vi "IviTriggerToProperty.vi"(8 "error in (no error)":errorcluster, 11 "IVI_Class.lvclass":refnum<class "IVI_Class.lvclass">) -> (0 "error out":errorcluster, 3 "IVI_Class.lvclass":refnum<class "IVI_Class.lvclass">)   [LabVIEW 2018, in "ScopePlugins.lvlib" / "IVI_Class.lvclass"]
doc: "Reads IVI Scope Acquisition properties and writes them into the Scope class Acquisition Properties"
uses:
  IVI_Class.lvclass
  C:/Users/ico/Documents/Projects/NistPluggableModules/Scope/ScopePlugins/ScopePluginBaseClass/ScopePluginsBase.lvclass
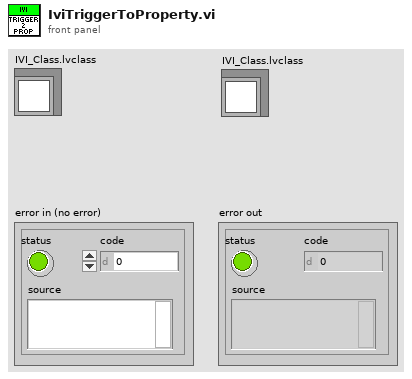
[diagram p1: front panel]
types:
  T1 = typedef "ScopePlugins.lvlib/ScopePluginsBase.lvclass/TriggerSettings.ctl" = cluster{"Common Trigger Settings":cluster{"Trigger Delay":dbl, "Reference Position":dbl, "Trigger Modifier":i32, "Auto Triggered":bool}, "Specific Trigger Settings":cluster{"Source":string, "Holdoff":dbl, "Level":dbl, "Trigger Slope":enum16{"Negative", "Positive"}, "Type":enum16{"Immediate", "Edge", "Digitial", "Window", "Hysteresis", "Width", "Runt", "Glitch", "TV", "AC Line"}, "Window Mode":i32, "Low Level":dbl, "High Level":dbl, "Coupling":u16, "Hysteresis":dbl}}
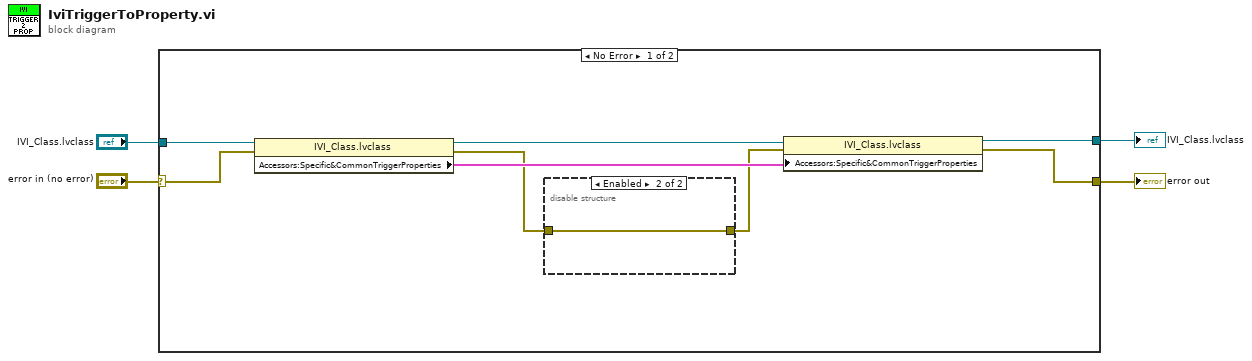
[diagram p0: block diagram]
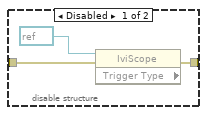
[diagram p2: hidden frame]
diagram:
  n1 = case shown="No Error" "error in (no error)" {
    selector: "error in (no error)" -> [w10 w17]
    tunnel: "IVI_Class.lvclass" -> [w12 w18]
    tunnel: [w11 w18] -> w3
    tunnel: [w9 w17] -> w1
    frame No Error {
      n2 = property class="IVI_Class.lvclass"(reference=w12, error in=w10) -> (reference out=w7:refnum<class "IVI_Class.lvclass">, error out=w6:errorcluster, "Accessors:Specific&CommonTriggerProperties"=w8:T1)
      n3 = disable-structure shown="Enabled" {
        disable-tunnel: [w15 w16] -> w5
        disable-tunnel: w6 -> [w13 w16]
        frame Disabled {
          n4 = property class="IviScope" props=["Trigger Type"](reference=refnum<k15> refnum ("reference out"), error in=w13) -> (error out=w15:errorcluster)  [unwired: 2 out]
        }
        frame Enabled {
        }
      }
      n5 = property class="IVI_Class.lvclass"(reference=w7, error in=w5, "Accessors:Specific&CommonTriggerProperties"=w8) -> (reference out=w11:refnum<class "IVI_Class.lvclass">, error out=w9:errorcluster)
    }
    frame Error {
    }
  }
  "IVI_Class.lvclass" <- w3
  "error out" <- w1
